vi "Event and Notifier Example.vi"() -> ()   [LabVIEW 2014]
uses:
  Type Definitions/UTILITY Notifier.ctl
panel:
  in  "Queue Set Status 2":bool
  in  "Queue Example Bool 2":bool
  in  "Event Stop":bool
  out "Numeric 6":i32
  out "Numeric 5":i32
  out "Event Stop":bool
  out "Queue Status":bool
  in  "error in (no error) 2":errorcluster
  out "error out 2":errorcluster
  out "latest READ notification 2":bool
  out "Numeric 4":i32
  out "Numeric 3":i32
  out "error out":errorcluster
  out "Queue Output":bool
  in  "Queue Stop":bool
  in  "Queue Set Status":bool
  in  "Queue Example Bool":bool
  in  "error in (no error)":errorcluster
  out "# elements in queue":i32
  out "Numeric 2":i32
  out "Numeric":i32
  in  "Exit Queue 2":bool
  out "element 2":bool
  in  "Send Noftify Queue 2":bool
  out "element":bool
  in  "Send Noftify Queue":bool
  in  "Exit Queue":bool
  in  "Exit Sub":bool
  out "latest READ notification":bool
  in  "Send Noftify Sub":bool
  in  "Exit Loop":bool
  out "notification":T1
  in  "Cluster 2":T1={"Numeric"=2.0, "Numeric 2"=0.0, "Boolean"=FALSE}
  in  "Cluster":T1
  in  "stop 4":bool
  in  "Event Stop":bool
  in  "stop 3":bool
  out "x+y":dbl
  in  "y":dbl
  in  "Send Notify":bool
  # "Notify Example 1"
  # "Notify Example 2"
  # "Queue Example 1"
  # "Queue Example 2"
  # "Event Example"
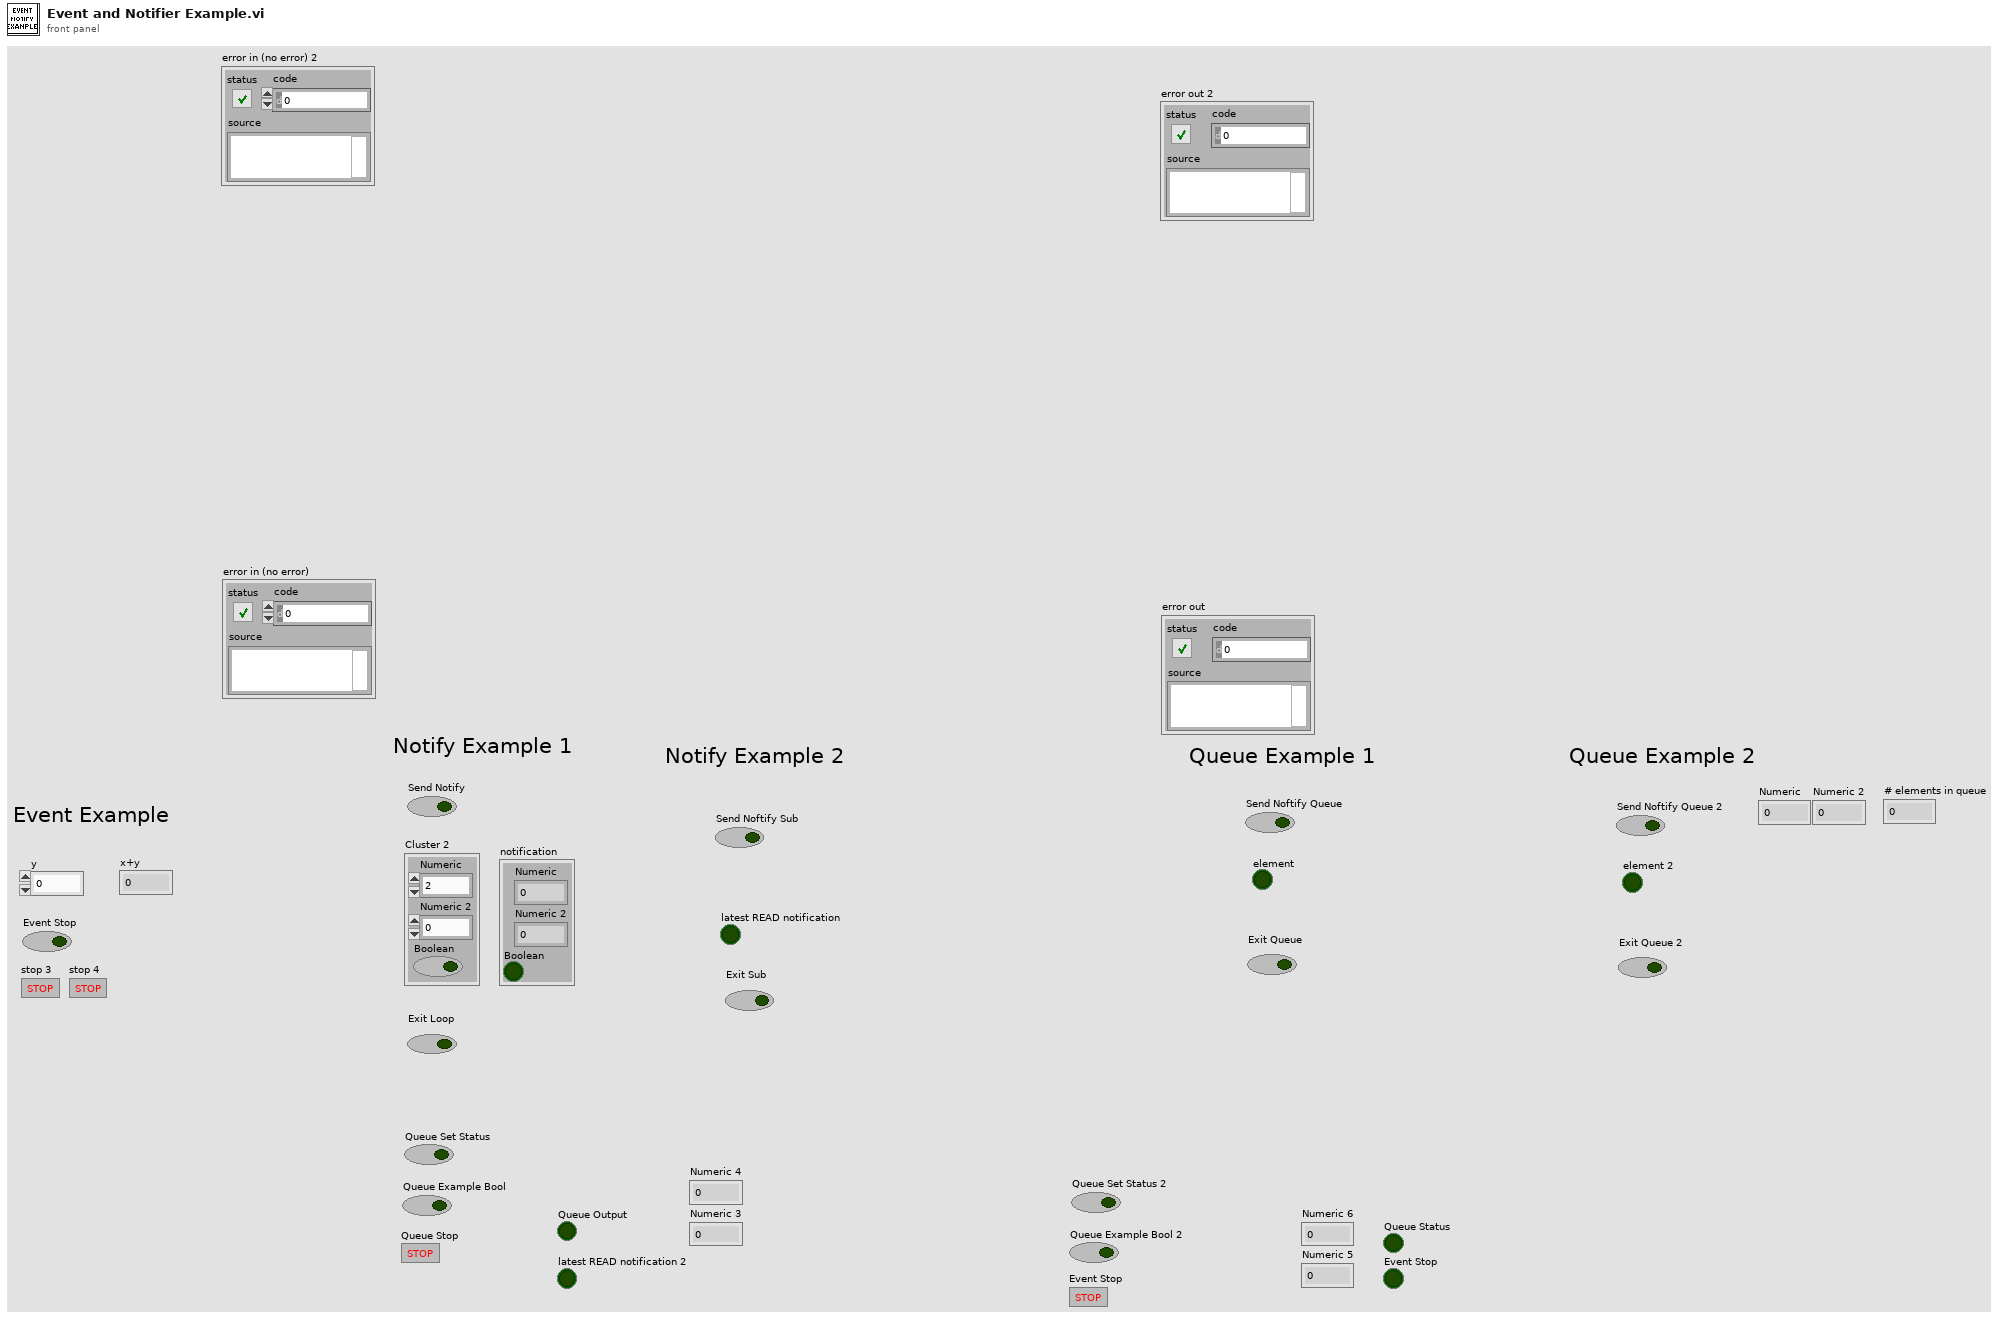
[diagram p1: front panel]
types:
  T1 = cluster{"Numeric":dbl, "Numeric 2":dbl, "Boolean":bool}
  T2 = typedef "UTILITY Notifier.ctl" = enum16{"Set", "Read", "Release Ref"}
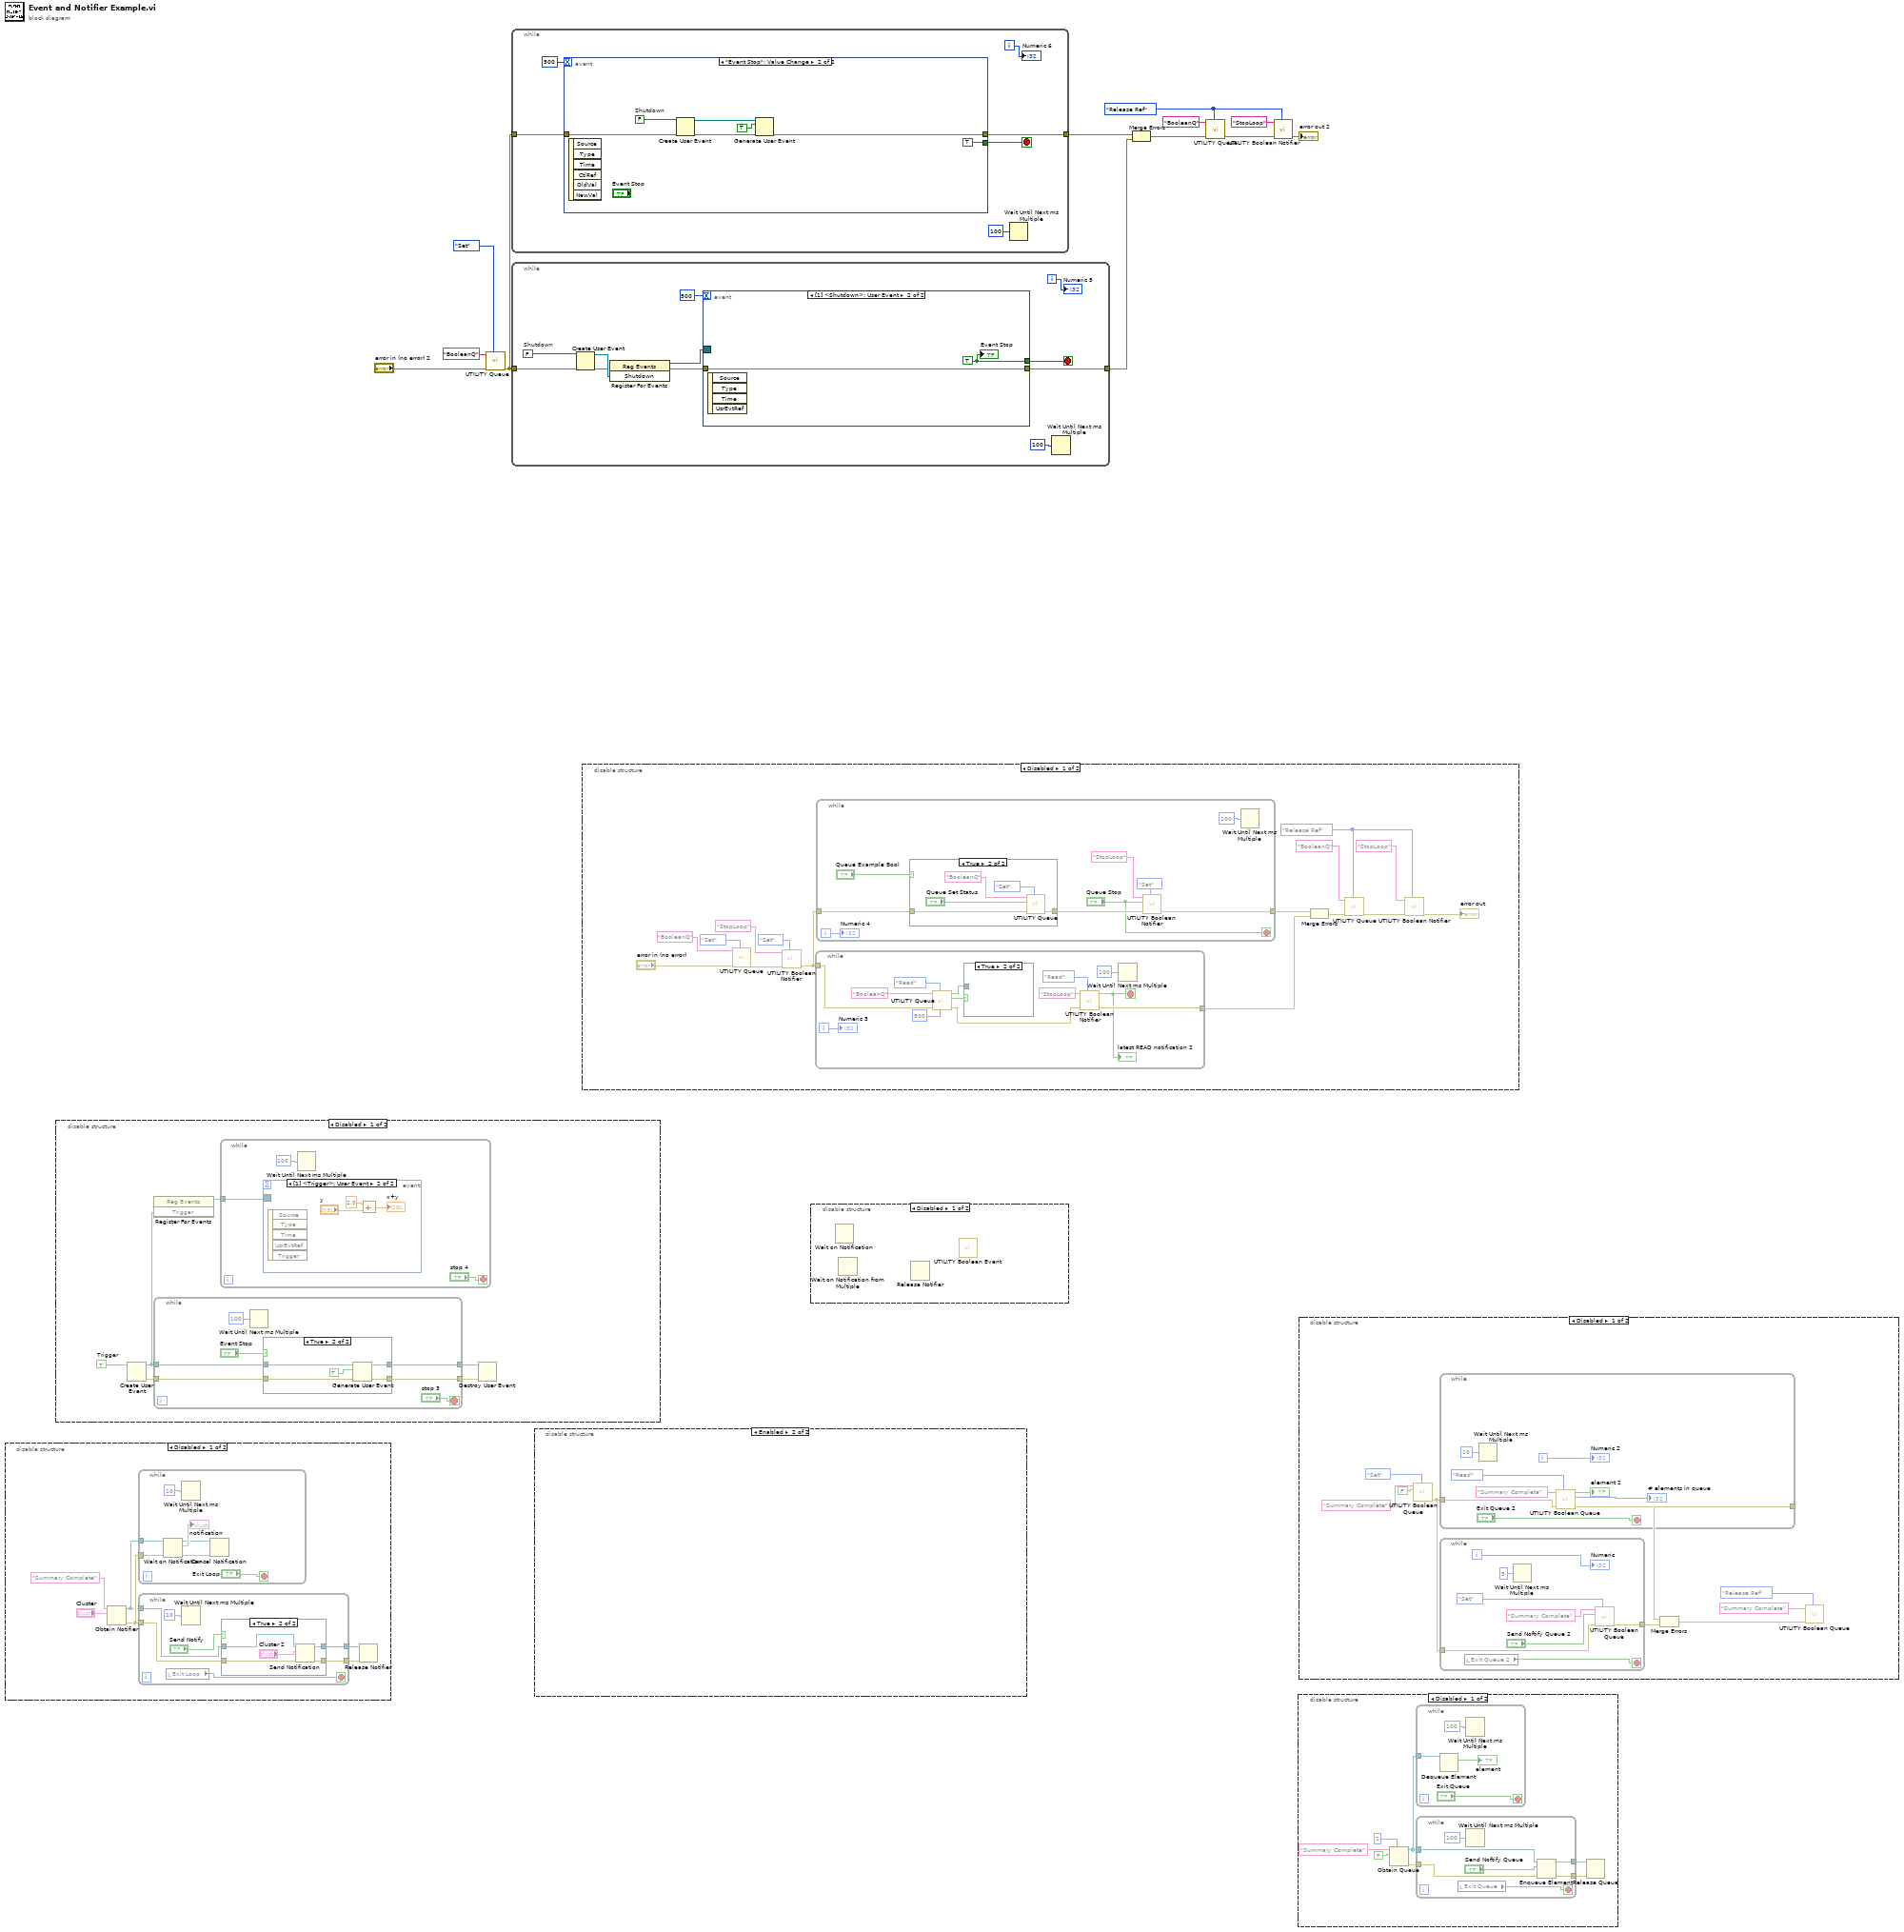
[diagram p0: block diagram]
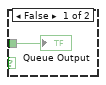
[diagram p2: hidden frame]
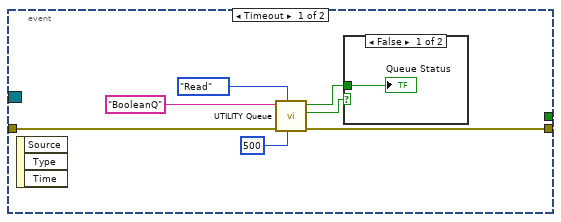
[diagram p5: hidden frame]
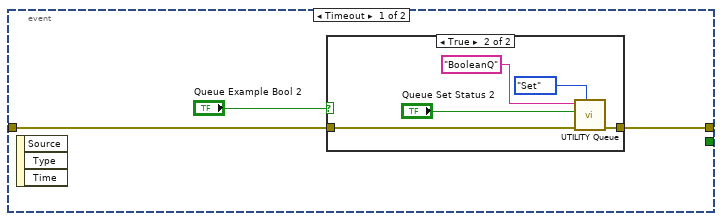
[diagram p7: hidden frame]
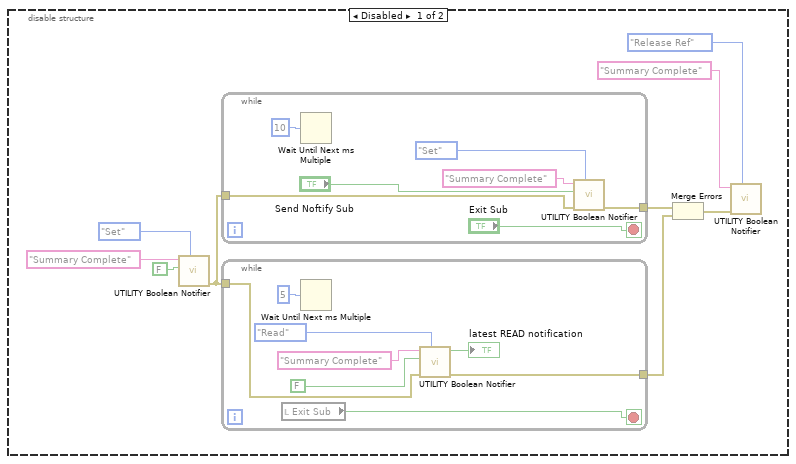
[diagram p11: hidden frame]
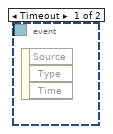
[diagram p15: hidden frame]
diagram:
  w11 = UTILITY_Notifier."Release Ref" ("Status")
  n1 = disable-structure shown="Disabled" {
    frame Disabled {
      n2 = Obtain Notifier(name (unnamed)="Summary Complete", notification data type="Cluster") -> (notifier out=w16:refnum<notifier>, error out=w17:errorcluster)  [unwired: 2 in, 1 out]
      n3 = while {
        tunnel: w17 -> [w25]
        tunnel: w16 -> [w24]
        stop <- "Exit Loop" stop-if-true
        n4 = Wait on Notification(notifier=w24, error in (no error)=w25) -> (notifier out=w19:refnum<notifier>, notification=→"notification":T1, error out=w20:errorcluster)  [unwired: 2 in, 1 out]
        n5 = Wait Until Next ms Multiple(millisecond multiple=u32 10) -> ()  [unwired: 1 out]
        n6 = Cancel Notification(0:w19, 3:w20) -> ()  [unwired: 3 out]
      }
      n7 = while {
        tunnel: w16 -> [w32]
        tunnel: w17 -> [w31]
        tunnel: [w30] -> w14
        tunnel: [w29] -> w15
        stop <- w26 stop-if-true
        n8 = local read "Exit Loop"() -> (w26:bool)
        n9 = Wait Until Next ms Multiple(millisecond multiple=u32 10) -> ()  [unwired: 1 out]
        n10 = case shown="True" "Send Notify" {
          tunnel: w32 -> [w34 w39]
          tunnel: w31 -> [w33 w38]
          tunnel: [w33 w37] -> w30
          tunnel: [w34 w36] -> w29
          frame False {
          }
          frame True {
            n11 = Send Notification(notification="Cluster 2", notifier=w39, error in (no error)=w38) -> (notifier out=w36:refnum<notifier>, error out=w37:errorcluster)
          }
        }
      }
      n12 = Release Notifier(notifier=w15, error in (no error)=w14) -> ()  [unwired: 1 in, 3 out]
    }
    frame Enabled {
    }
  }
  n13 = disable-structure shown="Disabled" {
    frame Disabled {
      w40 = TRUE  # Trigger
      n14 = Create User Event(user event datatype=w40) -> (user event=w44:refnum<user-event>, error out=w41:errorcluster)  [unwired: 1 in]
      n15 = register-events(w44) -> (reference out=w45:refnum<event-registration>)  [unwired: 2 in, 1 out]
      n16 = while {
        tunnel: w44 -> [w57]
        tunnel: w41 -> [w56]
        tunnel: [w55] -> w42
        tunnel: [w54] -> w43
        stop <- "stop 3" stop-if-true
        n17 = Wait Until Next ms Multiple(millisecond multiple=u32 100) -> ()  [unwired: 1 out]
        n18 = case shown="True" "Event Stop" {
          tunnel: w57 -> [w60 w65]
          tunnel: w56 -> [w59 w64]
          tunnel: [w59 w63] -> w55
          tunnel: [w60 w62] -> w54
          frame False {
          }
          frame True {
            n19 = Generate User Event(user event=w65, event data cluster=TRUE ("Trigger"), error in=w64) -> (user event out=w62:refnum<user-event>, error out=w63:errorcluster)  [unwired: 1 in]
          }
        }
      }
      n20 = while {
        tunnel: w45 -> [w48]
        stop <- "stop 4" stop-if-true
        n21 = event shown="[1] <Trigger>: User Event" {
          selector: w48 -> [_ _]
          dyn-events: _ -> [_ _]
          timeout: _ -> [_ _]
          event Timeout {
            n22 = event-data() -> ()  [unwired: 1 in, 3 out]
          }
          event User Event {
            n23 = event-data() -> ()  [unwired: 1 in, 5 out]
            n24 = Add(x=2.0, y="y") -> (x+y=→"x+y":dbl)
          }
        }
        n25 = Wait Until Next ms Multiple(millisecond multiple=u32 100) -> ()  [unwired: 1 out]
      }
      n26 = Destroy User Event(user event=w43, error in=w42) -> ()  [unwired: 1 out]
    }
    frame Enabled {
    }
  }
  n27 = call "UTILITY Queue.vi"("Status"=UTILITY_Notifier."Set", "error in (no error)"="error in (no error) 2", "name (unnamed)"="BooleanQ") -> ("error out"=w1:errorcluster)  [unwired: 6 in, 2 out]
  n28 = while {
    tunnel: w1 -> [w68]
    tunnel: [w67] -> w2
    i -> [w70]
    stop <- w69 stop-if-true
    n29 = event shown="[1] \"Event Stop\": Value Change" {
      selector: _ -> [_ _]
      dyn-events: _ -> [_ _]
      timeout: 500 -> [_ _]
      tunnel: w68 -> [w73 w83]
      tunnel: [_ TRUE] -> w69
      tunnel: [w72 w85] -> w67
      event Timeout {
        n30 = event-data() -> ()  [unwired: 1 in, 3 out]
        n31 = case shown="True" "Queue Example Bool 2" {
          tunnel: w73 -> [w75 w77]
          tunnel: [w75 w76] -> w72
          frame False {
          }
          frame True {
            n32 = call "UTILITY Queue.vi"("Status"=UTILITY_Notifier."Set", "error in (no error)"=w77, "Set Status"="Queue Set Status 2", "name (unnamed)"="BooleanQ") -> ("error out"=w76:errorcluster)  [unwired: 5 in, 2 out]
          }
        }
      }
      event "Event Stop": Value Change {
        w84 = FALSE  # Shutdown
        n33 = event-data() -> ()  [unwired: 1 in, 6 out]
        n34 = Create User Event(user event datatype=w84, error in=w83) -> (user event=w81:refnum<user-event>, error out=w82:errorcluster)
        n35 = Generate User Event(user event=w81, event data cluster=TRUE ("event data"), error in=w82) -> (error out=w85:errorcluster)  [unwired: 1 in, 1 out]
      }
    }
    n36 = Wait Until Next ms Multiple(millisecond multiple=u32 100) -> ()  [unwired: 1 out]
    "Numeric 6" <- w70
  }
  n37 = while {
    tunnel: w1 -> [w89]
    tunnel: [w95] -> w6
    i -> [w97]
    stop <- w96 stop-if-true
    w92 = FALSE  # Shutdown
    n38 = Create User Event(user event datatype=w92, error in=w89) -> (user event=w93:refnum<user-event>, error out=w90:errorcluster)
    n39 = register-events(error in=w90, w93) -> (reference out=w91:refnum<event-registration>, error out=w88:errorcluster)  [unwired: 1 in]
    n40 = event shown="[1] <Shutdown>: User Event" {
      selector: w91 -> [_ _]
      dyn-events: _ -> [_ _]
      timeout: 500 -> [_ _]
      tunnel: w88 -> [w100 w107]
      tunnel: [_ w108] -> w96
      tunnel: [w99 w107] -> w95
      event Timeout {
        n41 = event-data() -> ()  [unwired: 1 in, 3 out]
        n42 = call "UTILITY Queue.vi"("timeout in ms (-1)"=500, "Status"=UTILITY_Notifier."Read", "error in (no error)"=w100, "name (unnamed)"="BooleanQ") -> ("error out"=w99:errorcluster, "timed out?"=w101:bool, "latest READ notification"=w103:bool)  [unwired: 5 in]
        n43 = case shown="False" w101 {
          tunnel: w103 -> [w106 _]
          frame False {
            "Queue Status" <- w106
          }
          frame True {
          }
        }
      }
      event User Event {
        w108 = TRUE
        n44 = event-data() -> ()  [unwired: 1 in, 4 out]
        "Event Stop" <- w108
      }
    }
    n45 = Wait Until Next ms Multiple(millisecond multiple=u32 100) -> ()  [unwired: 1 out]
    "Numeric 5" <- w97
  }
  n46 = disable-structure shown="Enabled" {
    frame Disabled {
      n47 = call "UTILITY Boolean Notifier.vi"("Status"=UTILITY_Notifier."Set", "Set Status"=FALSE, "name (unnamed)"="Summary Complete") -> ("error out"=w114:errorcluster)  [unwired: 7 in, 1 out]
      n48 = while {
        tunnel: w114 -> [w132]
        tunnel: [w131] -> w113
        stop <- "Exit Sub" stop-if-true
        n49 = Wait Until Next ms Multiple(millisecond multiple=u32 10) -> ()  [unwired: 1 out]
        n50 = call "UTILITY Boolean Notifier.vi"("Status"=UTILITY_Notifier."Set", "error in (no error)"=w132, "Set Status"="Send Noftify Sub", "name (unnamed)"="Summary Complete") -> ("error out"=w131:errorcluster)  [unwired: 6 in, 1 out]
      }
      n51 = while {
        tunnel: w114 -> [w120]
        tunnel: [w119] -> w112
        stop <- w118 stop-if-true
        n52 = local read "Exit Sub"() -> (w118:bool)
        n53 = Wait Until Next ms Multiple(millisecond multiple=u32 5) -> ()  [unwired: 1 out]
        n54 = call "UTILITY Boolean Notifier.vi"("Status"=UTILITY_Notifier."Read", "error in (no error)"=w120, "Set Status"=FALSE, "name (unnamed)"="Summary Complete") -> ("error out"=w119:errorcluster, "latest READ notification"=→"latest READ notification":bool)  [unwired: 6 in]
      }
      n55 = Merge Errors(w113, w112) -> (w111:errorcluster)
      n56 = call "UTILITY Boolean Notifier.vi"("Status"=UTILITY_Notifier."Release Ref", "error in (no error)"=w111, "name (unnamed)"="Summary Complete") -> ()  [unwired: 7 in, 2 out]
    }
    frame Enabled {
    }
  }
  n57 = disable-structure shown="Disabled" {
    frame Disabled {
      w134 = UTILITY_Notifier."Release Ref" ("Status")
      n58 = call "UTILITY Queue.vi"("Status"=UTILITY_Notifier."Set", "error in (no error)"="error in (no error)", "name (unnamed)"="BooleanQ") -> ("error out"=w139:errorcluster)  [unwired: 6 in, 2 out]
      n59 = call "UTILITY Boolean Notifier.vi"("Status"=UTILITY_Notifier."Set", "error in (no error)"=w139, "name (unnamed)"="StopLoop") -> ("error out"=w137:errorcluster)  [unwired: 7 in, 1 out]
      n60 = while {
        tunnel: w137 -> [w150]
        tunnel: [w154] -> w143
        i -> [w156]
        stop <- w153 stop-if-true
        n61 = call "UTILITY Queue.vi"("timeout in ms (-1)"=500, "Status"=UTILITY_Notifier."Read", "error in (no error)"=w150, "name (unnamed)"="BooleanQ") -> ("error out"=w148:errorcluster, "timed out?"=w149:bool, "latest READ notification"=w158:bool)  [unwired: 5 in]
        n62 = case shown="True" w149 {
          tunnel: w158 -> [w161 _]
          frame False {
            "Queue Output" <- w161
          }
          frame True {
          }
        }
        n63 = call "UTILITY Boolean Notifier.vi"("Status"=UTILITY_Notifier."Read", "error in (no error)"=w148, "name (unnamed)"="StopLoop") -> ("error out"=w154:errorcluster, "latest READ notification"=w153:bool)  [unwired: 7 in]
        "latest READ notification 2" <- w153
        n64 = Wait Until Next ms Multiple(millisecond multiple=u32 100) -> ()  [unwired: 1 out]
        "Numeric 3" <- w156
      }
      n65 = while {
        tunnel: w137 -> [w168]
        tunnel: [w165] -> w144
        i -> [w167]
        stop <- "Queue Stop" stop-if-true
        n66 = case shown="True" "Queue Example Bool" {
          tunnel: w168 -> [w171 w173]
          tunnel: [w171 w172] -> w166
          frame False {
          }
          frame True {
            n67 = call "UTILITY Queue.vi"("Status"=UTILITY_Notifier."Set", "error in (no error)"=w173, "Set Status"="Queue Set Status", "name (unnamed)"="BooleanQ") -> ("error out"=w172:errorcluster)  [unwired: 5 in, 2 out]
          }
        }
        n68 = call "UTILITY Boolean Notifier.vi"("Status"=UTILITY_Notifier."Set", "error in (no error)"=w166, "Set Status"="Queue Stop", "name (unnamed)"="StopLoop") -> ("error out"=w165:errorcluster)  [unwired: 6 in, 1 out]
        n69 = Wait Until Next ms Multiple(millisecond multiple=u32 100) -> ()  [unwired: 1 out]
        "Numeric 4" <- w167
      }
      n70 = Merge Errors(w144, w143) -> (w142:errorcluster)
      n71 = call "UTILITY Queue.vi"("Status"=w134, "error in (no error)"=w142, "name (unnamed)"="BooleanQ") -> ("error out"=w136:errorcluster)  [unwired: 6 in, 2 out]
      n72 = call "UTILITY Boolean Notifier.vi"("Status"=w134, "error in (no error)"=w136, "name (unnamed)"="StopLoop") -> ("error out"=→"error out":errorcluster)  [unwired: 7 in, 1 out]
    }
    frame Enabled {
    }
  }
  n73 = disable-structure shown="Disabled" {
    frame Disabled {
      n74 = Wait on Notification() -> ()  [unwired: 4 in, 4 out]
      n75 = Wait on Notification from Multiple() -> ()  [unwired: 4 in, 4 out]
      n76 = Release Notifier() -> ()  [unwired: 3 in, 3 out]
      n77 = call "UTILITY Boolean Event.vi"() -> ()  [unwired: 10 in, 2 out]
    }
    frame Enabled {
    }
  }
  n78 = Merge Errors(w2, w6) -> (w7:errorcluster)
  n79 = call "UTILITY Queue.vi"("Status"=w11, "error in (no error)"=w7, "name (unnamed)"="BooleanQ") -> ("error out"=w9:errorcluster)  [unwired: 6 in, 2 out]
  n80 = call "UTILITY Boolean Notifier.vi"("Status"=w11, "error in (no error)"=w9, "name (unnamed)"="StopLoop") -> ("error out"=→"error out 2":errorcluster)  [unwired: 7 in, 1 out]
  n81 = disable-structure shown="Disabled" {
    frame Disabled {
      n82 = Obtain Queue(max queue size (-1, unlimited)=1, name (unnamed)="Summary Complete", element data type=FALSE ("Set Status")) -> (queue out=w181:refnum<queue>, error out=w178:errorcluster)  [unwired: 2 in, 1 out]
      n83 = while {
        tunnel: w181 -> [w192]
        stop <- "Exit Queue" stop-if-true
        n84 = Dequeue Element(queue=w192) -> (element=→"element":bool)  [unwired: 2 in, 3 out]
        n85 = Wait Until Next ms Multiple(millisecond multiple=u32 100) -> ()  [unwired: 1 out]
      }
      n86 = while {
        tunnel: w181 -> [w188]
        tunnel: [w186] -> w180
        tunnel: [w185] -> w179
        tunnel: w178 -> [w184]
        stop <- w190 stop-if-true
        n87 = local read "Exit Queue"() -> (w190:bool)
        n88 = Wait Until Next ms Multiple(millisecond multiple=u32 100) -> ()  [unwired: 1 out]
        n89 = Enqueue Element(queue=w188, element="Send Noftify Queue", error in (no error)=w184) -> (queue out=w186:refnum<queue>, error out=w185:errorcluster)  [unwired: 1 in, 1 out]
      }
      n90 = Release Queue(queue=w180, error in (no error)=w179) -> ()  [unwired: 1 in, 3 out]
    }
    frame Enabled {
    }
  }
  n91 = disable-structure shown="Disabled" {
    frame Disabled {
      n92 = call "UTILITY Boolean Queue.vi"("Status"=UTILITY_Notifier."Set", "Set Status"=FALSE, "name (unnamed)"="Summary Complete") -> ("error out"=w200:errorcluster)  [unwired: 6 in, 2 out]
      n93 = while {
        tunnel: w200 -> [w218]
        tunnel: [w214] -> w199
        i -> [w213]
        stop <- "Exit Queue 2" stop-if-true
        n94 = Wait Until Next ms Multiple(millisecond multiple=u32 10) -> ()  [unwired: 1 out]
        n95 = call "UTILITY Boolean Queue.vi"("Status"=UTILITY_Notifier."Read", "error in (no error)"=w218, "name (unnamed)"="Summary Complete") -> ("error out"=w214:errorcluster, "# elements in queue"=→"# elements in queue":i32, "latest READ notification"=→"element 2":bool)  [unwired: 6 in]
        "Numeric 2" <- w213
      }
      n96 = while {
        tunnel: [w208] -> w198
        tunnel: w200 -> [w206]
        i -> [w205]
        stop <- w211 stop-if-true
        n97 = local read "Exit Queue 2"() -> (w211:bool)
        n98 = Wait Until Next ms Multiple(millisecond multiple=u32 5) -> ()  [unwired: 1 out]
        n99 = call "UTILITY Boolean Queue.vi"("Status"=UTILITY_Notifier."Set", "error in (no error)"=w206, "Set Status"="Send Noftify Queue 2", "name (unnamed)"="Summary Complete") -> ("error out"=w208:errorcluster)  [unwired: 5 in, 2 out]
        "Numeric" <- w205
      }
      n100 = Merge Errors(w199, w198) -> (w197:errorcluster)
      n101 = call "UTILITY Boolean Queue.vi"("Status"=UTILITY_Notifier."Release Ref", "error in (no error)"=w197, "name (unnamed)"="Summary Complete") -> ()  [unwired: 6 in, 3 out]
    }
    frame Enabled {
    }
  }
